vi "FPGA main.vi"() -> ()   [LabVIEW 2012]
uses:
  <vilib>/rvi/Emulation/niFpgaSctlEmulationGetInTimedLoop.vi
  <vilib>/rvi/Emulation/niFpgaSctlEmulationGlobalWrite.vi
  <vilib>/rvi/eio/common/nirviEmuTemplateMethod_errors.vi
  <vilib>/eio/EIONode/EIONode.xnode
panel:
  out "结束标记":bool
  out "当前状态":i16
  out "parameter":i32
  out "开始标记":bool
  out "目标经度":i32
  in  "停止":bool
  out "当前经度":i32
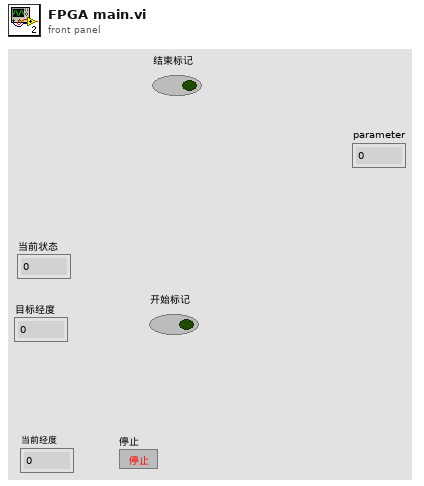
[diagram p1: front panel]
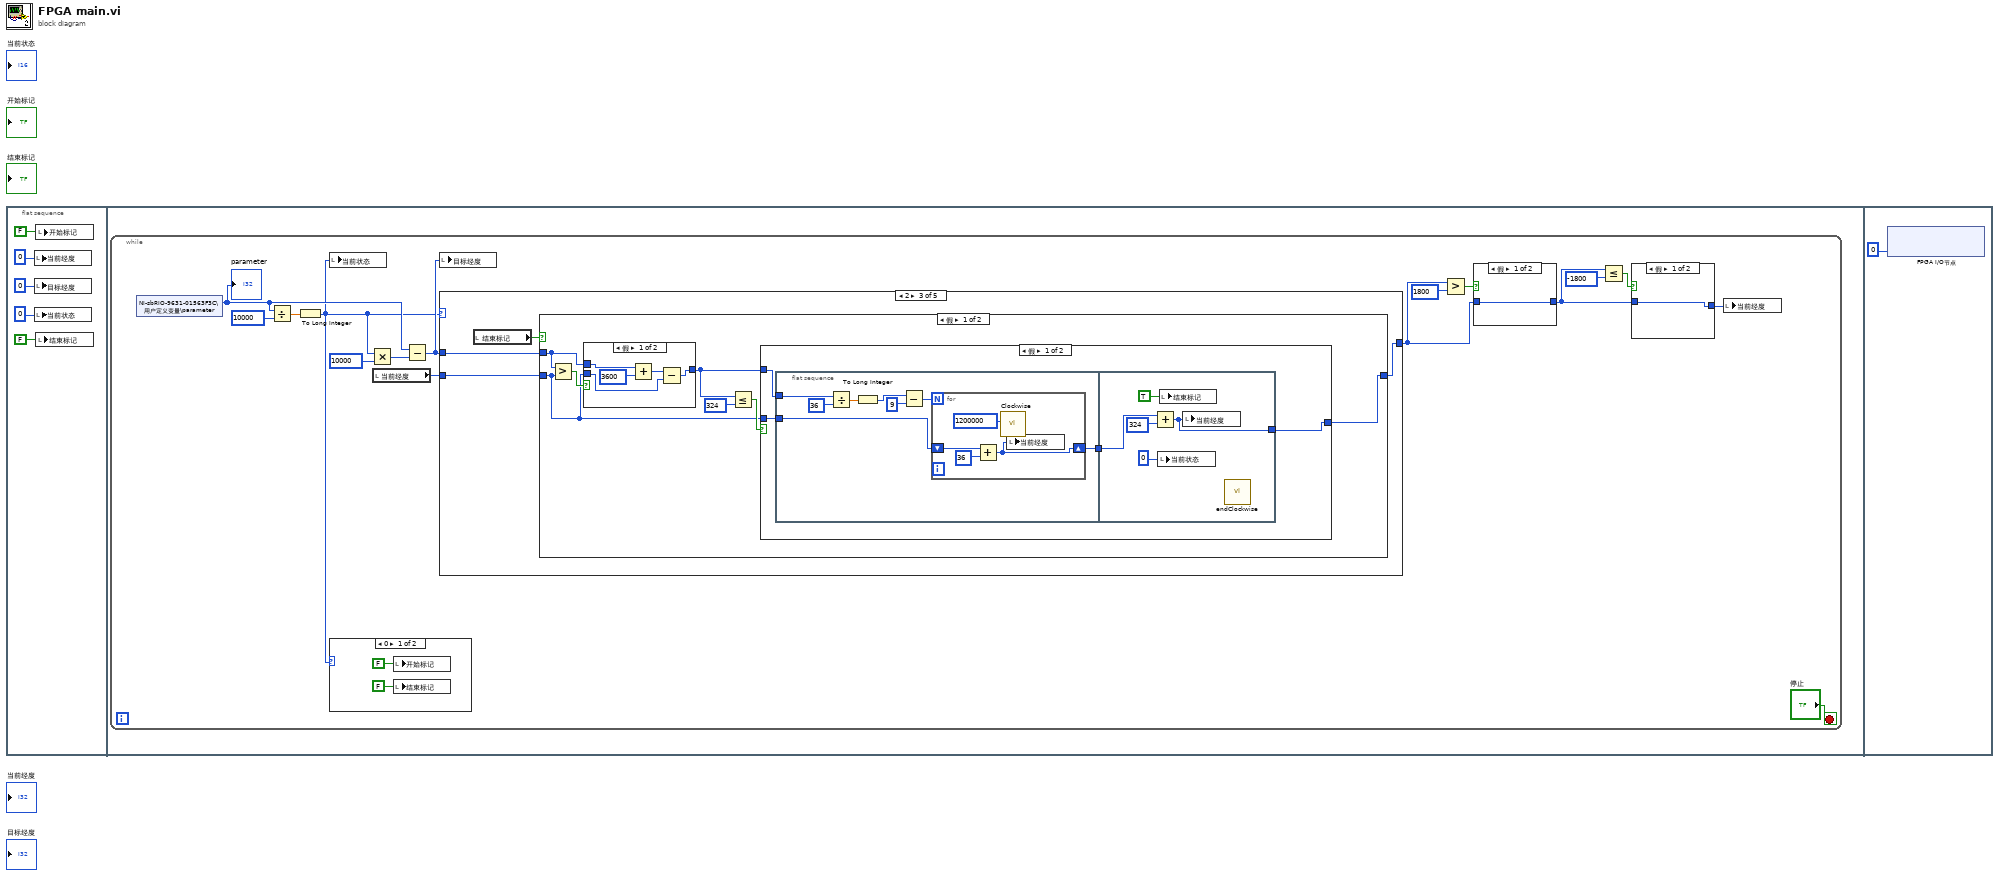
[diagram p0: block diagram]
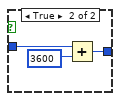
[diagram p2: hidden frame]
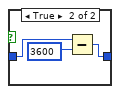
[diagram p3: hidden frame]
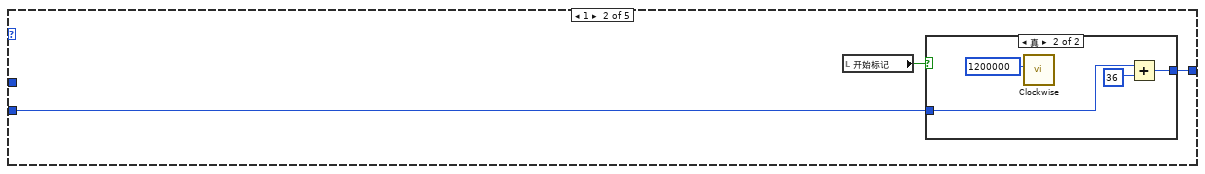
[diagram p6: hidden frame]
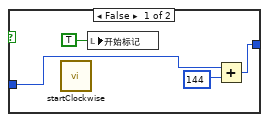
[diagram p7: hidden frame]
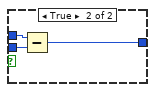
[diagram p8: hidden frame]
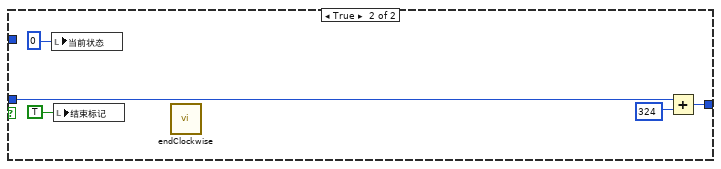
[diagram p9: hidden frame]
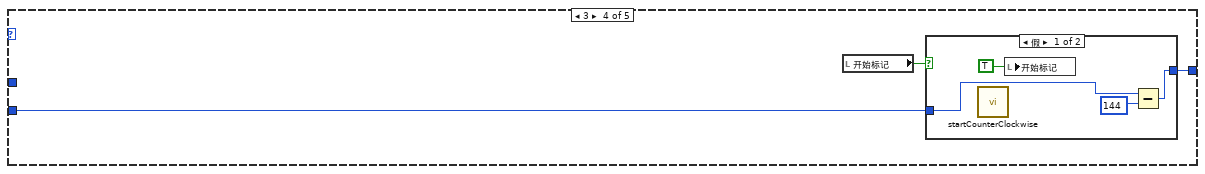
[diagram p11: hidden frame]
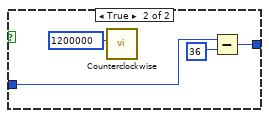
[diagram p12: hidden frame]
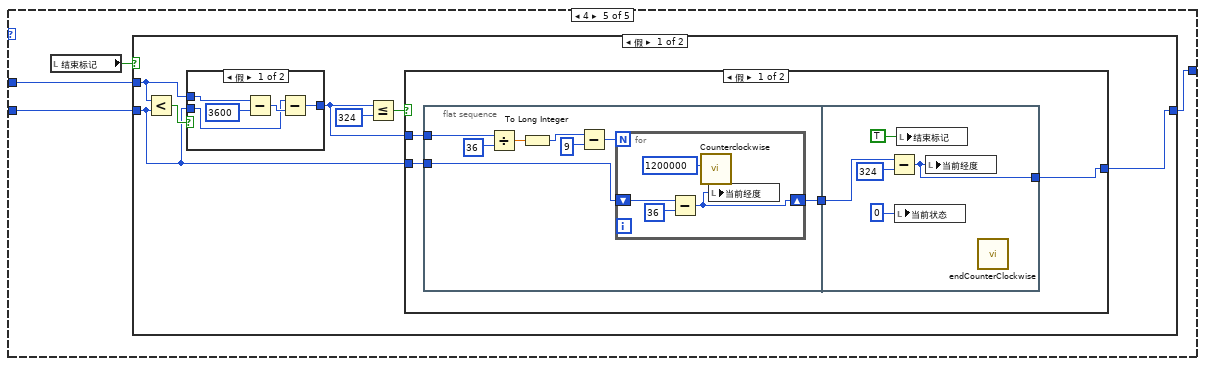
[diagram p13: hidden frame]
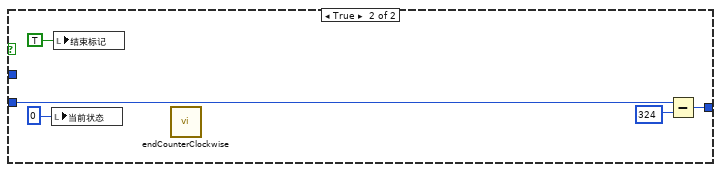
[diagram p14: hidden frame]
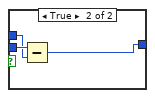
[diagram p15: hidden frame]
diagram:
  n1 = flat-sequence {
    frame #0 {
      n2 = local write "当前经度"(0 ("当前经度")) -> ()
      n3 = local write "目标经度"(0 ("目标经度")) -> ()
      n4 = local write "当前状态"(0 ("当前状态")) -> ()
      n5 = local write "开始标记"(FALSE ("开始标记")) -> ()
      n6 = local write "结束标记"(FALSE ("结束标记")) -> ()
    }
    frame #1 {
      n7 = while {
        stop <- "停止" stop-if-true
        n8 = shared-variable "NI-sbRIO-9631-01563F3C\\用户定义变量\\parameter"() -> (w18:i32)  [unwired: 1 in, 1 out]
        "parameter" <- w18
        n9 = Divide ("除")(x=w18, y=10000) -> (x/y=w19:sgl)
        n10 = To Long Integer(number=w19) -> (32bit integer=w6:i32)
        n11 = local write "当前状态"(w6) -> ()
        n12 = case shown="0" w6 {
          frame 0 {
            n13 = local write "开始标记"(FALSE ("开始标记")) -> ()
            n14 = local write "结束标记"(FALSE ("结束标记")) -> ()
          }
          frame 1, Default {
          }
        }
        n15 = Multiply(x=w6, y=10000) -> (x*y=w16:i32)
        n16 = local read "当前经度"() -> (w14:i32)
        n17 = Subtract(x=w18, y=w16) -> (x-y=w7:i32)
        n18 = local write "目标经度"(w7) -> ()
        n19 = case shown="2" w6 {
          tunnel: w14 -> [w32 w34 w46 w91 w103]
          tunnel: [w32 w33 w44 w90 w101] -> w15
          tunnel: w7 -> [_ _ w45 _ w102]
          frame 0, Default {
          }
          frame 1 {
            n20 = local read "开始标记"() -> (w35:bool)
            n21 = case shown="真" w35 {
              tunnel: w34 -> [w37 w41]
              tunnel: [w36 w40] -> w33
              frame False {
                n22 = call "startClockwise.vi"() -> ()  [unwired: 12 in]
                n23 = local write "开始标记"(TRUE ("开始标记")) -> ()
                n24 = Add(x=w37, y=144) -> (x+y=w36:i32)
              }
              frame True {
                n25 = call "Clockwise.vi"("Count(Ticks)"=u32 1200000) -> ()  [unwired: 11 in]
                n26 = Add(x=w41, y=36) -> (x+y=w40:i32)
              }
            }
          }
          frame 2 {
            n27 = local read "结束标记"() -> (w47:bool)
            n28 = case shown="假" w47 {
              tunnel: w46 -> [w50 w89]
              tunnel: w45 -> [w49 _]
              tunnel: [w48 w89] -> w44
              frame False {
                n29 = Greater?(x=w49, y=w50) -> (0:w54:bool)
                n30 = case shown="假" w54 {
                  tunnel: w49 -> [w59 w62]
                  tunnel: w50 -> [w56 w61]
                  tunnel: [w55 w60] -> w51
                  frame False {
                    n31 = Add(x=w59, y=3600) -> (x+y=w57:i32)
                    n32 = Subtract(x=w57, y=w56) -> (x-y=w55:i32)
                  }
                  frame True {
                    n33 = Subtract(x=w62, y=w61) -> (x-y=w60:i32)
                  }
                }
                n34 = Less Or Equal?(x=w51, y=324) -> (x <= y?=w52:bool)
                n35 = case shown="假" w52 {
                  tunnel: w51 -> [w66 _]
                  tunnel: w50 -> [w65 w87]
                  tunnel: [w63 w86] -> w48
                  frame False {
                    n36 = flat-sequence {
                      tunnel: w66 -> [w73]
                      tunnel: w65 -> [w71]
                      tunnel: [w70] -> w64
                      tunnel: w64 -> [w82]
                      tunnel: [w79] -> w63
                      frame #0 {
                        n37 = Divide ("除")(x=w73, y=36) -> (x/y=w72:sgl)
                        n38 = To Long Integer(number=w72) -> (32bit integer=w69:i32)
                        n39 = Subtract(x=w69, y=9) -> (x-y=w67:i32)
                        n40 = for {
                          N: w67 -> [_]
                          shift-right: [w75] -> w70
                          shift-left: w71 -> [w76]
                          n41 = Add(x=w76, y=36) -> (x+y=w75:i32)
                          n42 = call "Clockwise.vi"("Count(Ticks)"=u32 1200000) -> ()  [unwired: 11 in]
                          n43 = local write "当前经度"(w75) -> ()
                        }
                      }
                      frame #1 {
                        n44 = Add(x=w82, y=324) -> (x+y=w79:i32)
                        n45 = local write "当前状态"(i16 0 ("当前状态")) -> ()
                        n46 = local write "结束标记"(TRUE ("结束标记")) -> ()
                        n47 = local write "当前经度"(w79) -> ()
                        n48 = call "endClockwise.vi"() -> ()  [unwired: 12 in]
                      }
                    }
                  }
                  frame True {
                    n49 = local write "当前状态"(i16 0 ("当前状态")) -> ()
                    n50 = local write "结束标记"(TRUE ("结束标记")) -> ()
                    n51 = call "endClockwise.vi"() -> ()  [unwired: 12 in]
                    n52 = Add(x=w87, y=324) -> (x+y=w86:i32)
                  }
                }
              }
              frame True {
              }
            }
          }
          frame 3 {
            n53 = local read "开始标记"() -> (w92:bool)
            n54 = case shown="假" w92 {
              tunnel: w91 -> [w94 w98]
              tunnel: [w93 w97] -> w90
              frame False {
                n55 = call "startCounterClockwise.vi"() -> ()  [unwired: 12 in]
                n56 = local write "开始标记"(TRUE ("开始标记")) -> ()
                n57 = Subtract(x=w94, y=144) -> (x-y=w93:i32)
              }
              frame True {
                n58 = call "Counterclockwise.vi"("Count(Ticks)"=u32 1200000) -> ()  [unwired: 11 in]
                n59 = Subtract(x=w98, y=36) -> (x-y=w97:i32)
              }
            }
          }
          frame 4 {
            n60 = local read "结束标记"() -> (w104:bool)
            n61 = case shown="假" w104 {
              tunnel: w103 -> [w107 w146]
              tunnel: w102 -> [w106 _]
              tunnel: [w105 w146] -> w101
              frame False {
                n62 = Less?(x=w106, y=w107) -> (x < y?=w111:bool)
                n63 = case shown="假" w111 {
                  tunnel: w107 -> [w139 w145]
                  tunnel: w106 -> [w142 w144]
                  tunnel: [w138 w143] -> w108
                  frame False {
                    n64 = Subtract(x=w142, y=3600) -> (x-y=w140:i32)
                    n65 = Subtract(x=w139, y=w140) -> (x-y=w138:i32)
                  }
                  frame True {
                    n66 = Subtract(x=w145, y=w144) -> (x-y=w143:i32)
                  }
                }
                n67 = Less Or Equal?(x=w108, y=324) -> (x <= y?=w109:bool)
                n68 = case shown="假" w109 {
                  tunnel: w108 -> [w115 _]
                  tunnel: w107 -> [w114 w136]
                  tunnel: [w112 w133] -> w105
                  frame False {
                    n69 = flat-sequence {
                      tunnel: w115 -> [w123]
                      tunnel: w114 -> [w120]
                      tunnel: [w119] -> w113
                      tunnel: w113 -> [w131]
                      tunnel: [w128] -> w112
                      frame #0 {
                        n70 = Divide ("除")(x=w123, y=36) -> (x/y=w121:sgl)
                        n71 = To Long Integer(number=w121) -> (32bit integer=w118:i32)
                        n72 = Subtract(x=w118, y=9) -> (x-y=w116:i32)
                        n73 = for {
                          N: w116 -> [_]
                          shift-right: [w124] -> w119
                          shift-left: w120 -> [w125]
                          n74 = Subtract(x=w125, y=36) -> (x-y=w124:i32)
                          n75 = call "Counterclockwise.vi"("Count(Ticks)"=u32 1200000) -> ()  [unwired: 11 in]
                          n76 = local write "当前经度"(w124) -> ()
                        }
                      }
                      frame #1 {
                        n77 = Subtract(x=w131, y=324) -> (x-y=w128:i32)
                        n78 = local write "当前状态"(i16 0 ("当前状态")) -> ()
                        n79 = local write "结束标记"(TRUE ("结束标记")) -> ()
                        n80 = local write "当前经度"(w128) -> ()
                        n81 = call "endCounterClockwise.vi"() -> ()  [unwired: 12 in]
                      }
                    }
                  }
                  frame True {
                    n82 = local write "当前状态"(i16 0 ("当前状态")) -> ()
                    n83 = local write "结束标记"(TRUE ("结束标记")) -> ()
                    n84 = call "endCounterClockwise.vi"() -> ()  [unwired: 12 in]
                    n85 = Subtract(x=w136, y=324) -> (x-y=w133:i32)
                  }
                }
              }
              frame True {
              }
            }
          }
        }
        n86 = Greater?(x=w15, y=1800) -> (0:w12:bool)
        n87 = case shown="假" w12 {
          tunnel: w15 -> [w26 w29]
          tunnel: [w26 w27] -> w9
          frame False {
          }
          frame True {
            n88 = Subtract(x=w29, y=3600) -> (x-y=w27:i32)
          }
        }
        n89 = Less Or Equal?(x=w9, y=-1800) -> (x <= y?=w11:bool)
        n90 = case shown="假" w11 {
          tunnel: w9 -> [w22 w25]
          tunnel: [w22 w23] -> w8
          frame False {
          }
          frame True {
            n91 = Add(x=w25, y=3600) -> (x+y=w23:i32)
          }
        }
        n92 = local write "当前经度"(w8) -> ()
      }
    }
    frame #2 {
      n93 = xnode "FPGA I/O节点"("Port6/DIO9:0"=i8 0 ("IO")) -> ()  [unwired: 1 in, 1 out]
    }
  }
